vi "nirvimemoryPaletteMergeVI.vi"   [LabVIEW 2017]
doc: "Invokes a method on a memory block on the FPGA. The methods available depend on the type of memory you configure.\n\nYou must specify a memory item before you specify a method.\n\nYou can invoke the following memory methods for memory you implement as block memory or look-up tables:\n\nWrite\n\nRead\n\nYou can invoke the following memory methods for memory you implement as DRAM:\n\nWrite\n\nRequest Data\n\nRetrieve Data\n\n<B>Note</B> When you configure the memory to have two read interfaces, the Read method contains an <B>[A]</B> or <B>[B]</B> in the label to denote which interface the node will access."
uses:
  <vilib>/rvi/DataTransferAndStorage/Container/XNode/niFpgaContainer.xnode
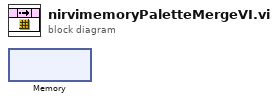
[diagram p0: block diagram]
diagram:
  n1 = xnode "Memory"() -> ()  [unwired: 1 in, 1 out]
